vi "Loop for.vi"() -> ()   [LabVIEW 2024]
panel:
  in  "Alavanca":bool
  out "Saída":dbl[](array[numeric])
  out "Boolean":bool
  out "String":string
  in  "N Value":dbl
  out "Progress Bar":dbl(slide) scale=0.0..200.0
  in  "Array 2 - 0":dbl
  in  "Array 2 - 1":dbl
  out "I Value":i32
  in  "Array 1 - 1":dbl
  in  "Array 1 - 0":dbl
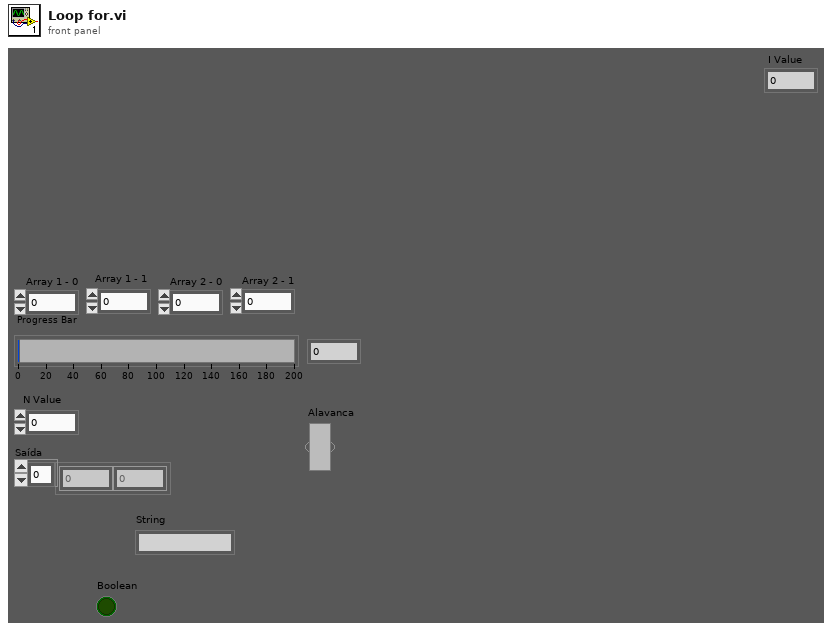
[diagram p1: front panel]
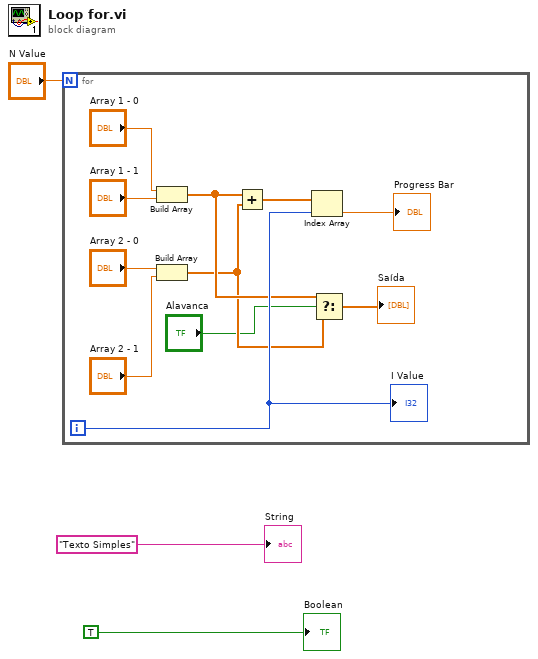
[diagram p0: block diagram]
diagram:
  n1 = for {
    N: "N Value" -> [_]
    i -> [w9]
    n2 = Build Array("Array 1 - 0", "Array 1 - 1") -> (w7:dbl[])
    n3 = Build Array("Array 2 - 0", "Array 2 - 1") -> (w6:dbl[])
    n4 = Add(x=w7, y=w6) -> (x+y=w10:dbl[])
    n5 = Index Array(array=w10, index=w9) -> (element=→"Progress Bar":dbl)
    n6 = Select(t=w7, s="Alavanca", f=w6) -> (s? t:f=→"Saída":dbl[])
    "I Value" <- w9
  }
  "String" <- "Texto Simples" ("String")
  "Boolean" <- TRUE
